vi "RF Traces to Intensity Plots.vi"(8 "Error In":errorcluster, 9 "Waveforms In":waveform(dbl)[](array[waveform]), 10 "Channel":i32) -> (0 "Error Out":errorcluster, 1 "Intensity Out [dB]":dbl[][](array[numeric]), 2 "Wavefronts":dbl[][](array[numeric]), 3 "Intensity Chart xy Scale":T1, 4 "t0":timestamp)   [LabVIEW 2019]
uses:
  Controls/Intensity Chart Scale.ctl
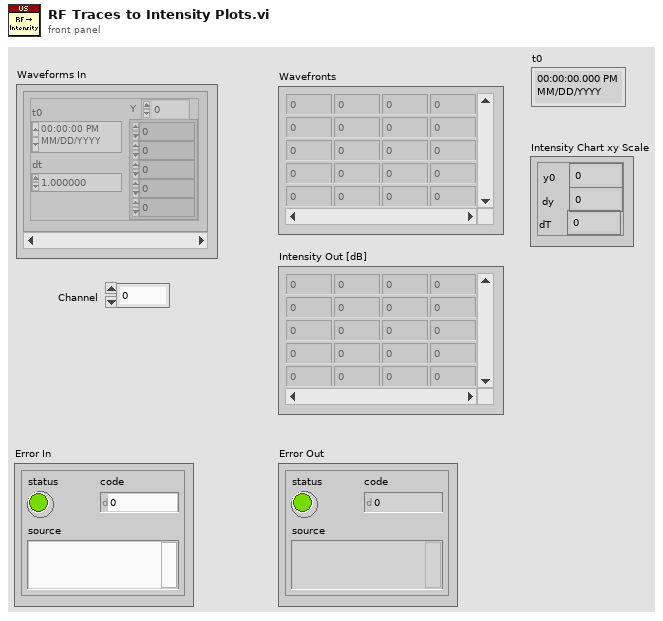
[diagram p1: front panel]
types:
  T1 = typedef "Intensity Chart Scale.ctl" = cluster{"y0":dbl, "dy":dbl, "dT":dbl}
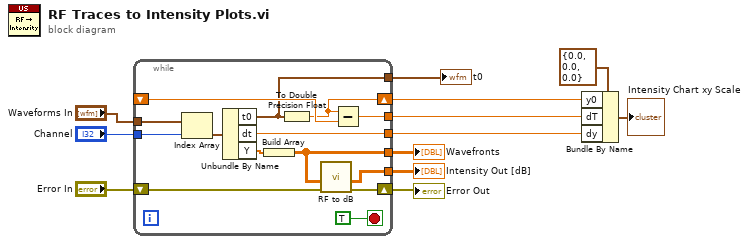
[diagram p0: block diagram]
diagram:
  n1 = while {
    tunnel: "Channel" -> [w24]
    tunnel: "Waveforms In" -> [w23]
    tunnel: [w22] -> w10
    tunnel: [w21] -> w9
    tunnel: [w18] -> w4
    shift-right: [w19] -> w7
    shift-left: "Error In" -> [w20]
    shift-right: [w14] -> w3
    shift-left: _ -> [w16]
    tunnel: [w15] -> w5
    tunnel: [w13] -> w2
    stop <- TRUE stop-if-true
    n2 = Index Array(array=w23, index=w24) -> (element=w26:waveform(dbl))
    n3 = Unbundle By Name(w26) -> ("t0"=w13:timestamp, "dt"=w18:dbl, "Y"=w25:dbl[])
    n4 = Build Array(w25) -> (w22:dbl[][])
    n5 = To Double Precision Float(number=w13) -> (double precision float=w14:dbl)
    n6 = call "RF to dB.vi"("Error In"=w20, "RF"=w22) -> ("Error Out"=w19:errorcluster, "dB"=w21:dbl[][])  [unwired: 8 in]
    n7 = Subtract(x=w14, y=w16) -> (x-y=w15:dbl)
  }
  "Wavefronts" <- w10
  "Intensity Out [dB]" <- w9
  "Error Out" <- w7
  "t0" <- w2
  n8 = Bundle By Name(cluster=T1 {"y0"=0.0, "dy"=0.0, "dT"=0.0} ("Intensity Chart Scale"), "y0"=w3, "dT"=w5, "dy"=w4) -> (→"Intensity Chart xy Scale":T1)
